vi "AB_Log_Destinations.vi"(8 "error in (no error)":errorcluster, 11 "destinations":refnum<class "AB_Destination.lvclass">[](array[class])) -> (0 "error out":errorcluster)   [LabVIEW 2020]
uses:
  <vilib>/AppBuilder/AB_Classes/Destination/AB_Destination.lvclass
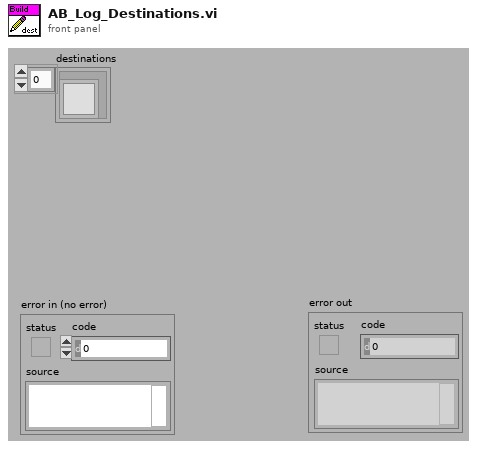
[diagram p1: front panel]
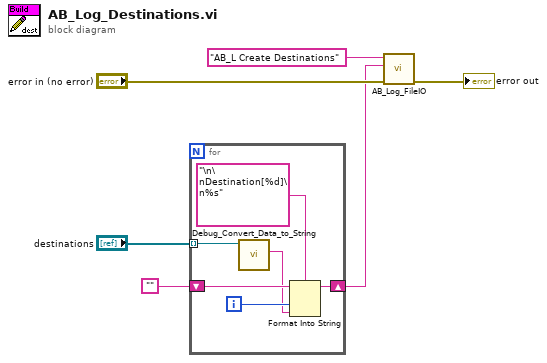
[diagram p0: block diagram]
diagram:
  n1 = for {
    shift-right: [w10] -> w4
    shift-left: "" -> [w11]
    tunnel: "destinations" -> [w8] mode=indexing
    i -> [w9]
    n2 = call-dynamic "Debug_Convert_Data_to_String.vi"("AB_Destination in"=w8) -> ("classData"=w7:string)  [unwired: 8 in, 2 out]
    n3 = Format Into String(format string="\n\nDestination[%d]\n%s", initial string=w11, w9, w7) -> (resulting string=w10:string)  [unwired: 1 in, 1 out]
  }
  n4 = call <vilib>:"AB_Log_FileIO.vi"("error in (no error)"="error in (no error)", "data"=w4, "newSection"="AB_L Create Destinations") -> ("error out"=→"error out":errorcluster)  [unwired: 8 in]
